vi "render_overlay_guide_horizontal.vi"(4 "ROI":i32[](array[numeric]), 5 "Group":string, 8 "Position (real coords)":dbl, 9 "Image":T1) -> (3 "Image Out":T1)   [LabVIEW 2019]
uses:
  <vilib>/vision/Image Controls.llb/IMAQ Image.ctl
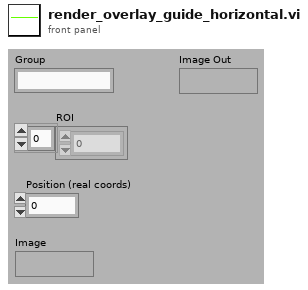
[diagram p1: front panel]
types:
  T1 = typedef "IMAQ Image.ctl" = refnum<image>
  T2 = cluster{"Grid Spacing":dbl, "Position (real coords)":dbl, "Grid Spacing":dbl}
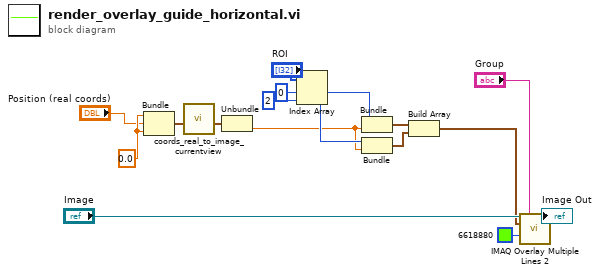
[diagram p0: block diagram]
diagram:
  w4 = 0.0 ("Grid Spacing")
  n1 = Bundle("Grid Spacing"=w4, "Position (real coords)"="Position (real coords)", "Grid Spacing"=w4) -> (w7:T2)  [unwired: 1 in]
  n2 = call "coords_real_to_image_currentview.vi"("Position (real coords)"=w7) -> ("Position (pixels, relative to the top left of the image)"=w1:cluster{dbl, dbl})  [unwired: 7 in, 1 out]
  n3 = Unbundle(w1) -> (w2:dbl)  [unwired: 1 out]
  n4 = Index Array(array="ROI", index #1=0 ("index"), index #2=2 ("index")) -> (element #1=w6:i32, element #2=w5:i32)
  n5 = Bundle("Numeric"=w6, w2) -> (w11:cluster{"Numeric":i32, dbl})  [unwired: 1 in]
  n6 = Bundle("Numeric"=w5, w2) -> (w12:cluster{"Numeric":i32, dbl})  [unwired: 1 in]
  n7 = Build Array(w11, w12) -> (w13:cluster{"Numeric":i32, dbl}[])
  n8 = call "IMAQ Overlay Multiple Lines 2"("Image"="Image", "Group"="Group", "Line End Points"=w13, "Color"=u32 6618880) -> ("Image Out"=→"Image Out":T1)  [unwired: 10 in, 1 out]
